vi "1BLABVIEW.vi"() -> ()   [LabVIEW 2013]
panel:
  out "NAND":bool
  out "XOR":bool
  out "NOT":bool
  out "OR":bool
  out "AND":bool
  in  "B":bool
  in  "A":bool
  # "1(b).LOGIC GATES"
  # "O.SRINIVAS\n23A91A04H6"
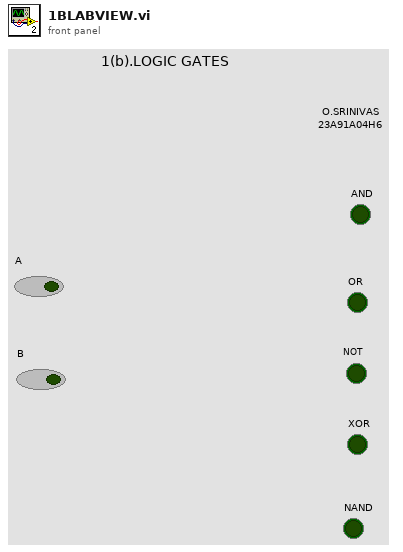
[diagram p1: front panel]
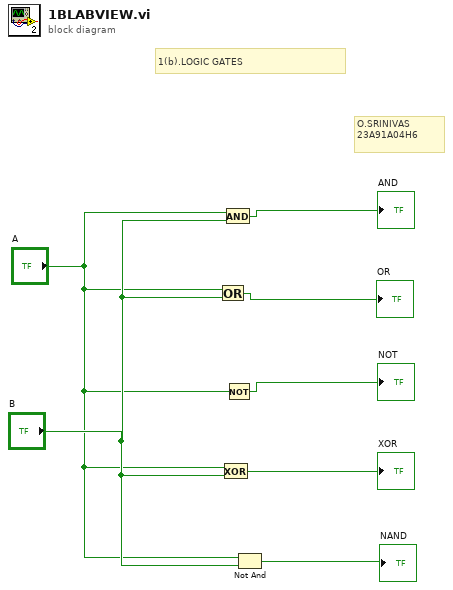
[diagram p0: block diagram]
diagram:
  # "O.SRINIVAS\n23A91A04H6"
  # "1(b).LOGIC GATES"
  n1 = Or(x="A", y="B") -> (x .or. y?=→"OR":bool)
  n2 = Exclusive Or(1:"B", 2:"A") -> (0:→"XOR":bool)
  n3 = And(x="A", y="B") -> (x .and. y?=→"AND":bool)
  n4 = Not(x="A") -> (.not. x?=→"NOT":bool)
  n5 = Not And(1:"B", 2:"A") -> (0:→"NAND":bool)
